vi "Request Data.vi"(6 "Qualifier":string, 8 "error in":errorcluster, 9 "notifier":refnum<notifier>, 10 "Data to Send":string, 11 "MLTFNC in":refnum<class "MLTFNC.lvclass">) -> (0 "error out":errorcluster, 3 "MLTFNC out":refnum<class "MLTFNC.lvclass">)   [LabVIEW 2019, in "MLTFNC.lvlib" / "MLTFNC.lvclass"]
doc: "Data to Send is a required input that describes the measurement or query function to be performed\nQualifier is a secondary variable used in the event that specificity must be provided to the query function\n****Note****\nIf further specificity is required, the qualifier must be used in a comma delimited format to increase the overall variable count. Additional specificity must be provided by the child class and interpreted by the automated call.\n\nnotifier is a single variant notifier in which the instrument will send the data notification to the automated tool."
uses:
  Library/MLTFNC.lvclass
  C:/Users/Public/Documents/Development/builds/Instruments/Instruments.lvlibp/Library/Instruments.lvclass
  builds/Instruments/Instruments.lvlibp/Private/Accessors/Read Poll(ms).vi
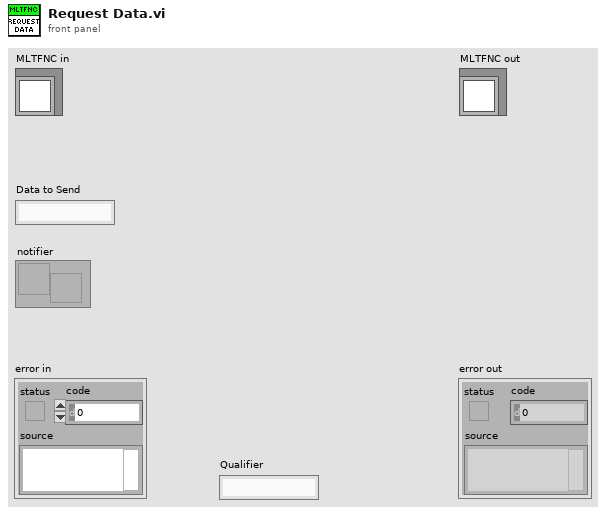
[diagram p1: front panel]
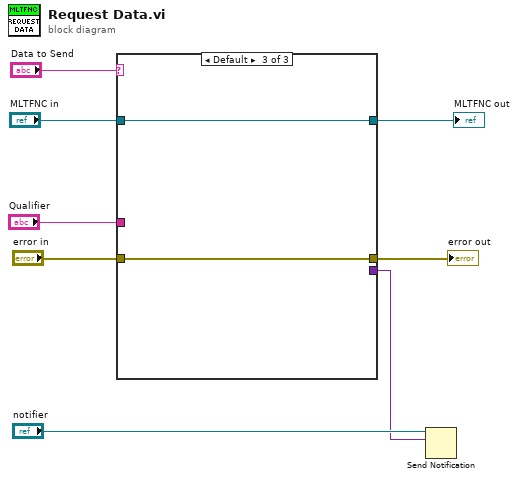
[diagram p0: block diagram]
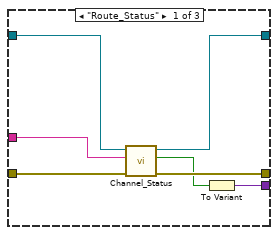
[diagram p2: hidden frame]
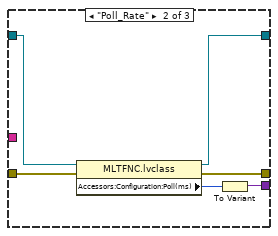
[diagram p3: hidden frame]
diagram:
  n1 = case shown="Default" "Data to Send" {
    tunnel: "MLTFNC in" -> [w15 w19 w23]
    tunnel: [w14 w18 w23] -> w6
    tunnel: "error in" -> [w12 w21 w22]
    tunnel: [w11 w20 w22] -> w3
    tunnel: "Qualifier" -> [w13 _ _]
    tunnel: [w9 w16 _] -> w1
    frame "Route_Status" {
      n2 = call "Channel_Status.vi"("error in"=w12, "Channel"=w13, "MLTFNC in"=w15) -> ("error out"=w11:errorcluster, "Routed"=w10:bool, "MLTFNC out"=w14:refnum<class "MLTFNC.lvclass">)  [unwired: 6 in]
      n3 = To Variant(anything=w10) -> (Variant=w9:variant)
    }
    frame "Poll_Rate" {
      n4 = property class="MLTFNC.lvclass"(reference=w19, error in=w21) -> (reference out=w18:refnum<class "MLTFNC.lvclass">, error out=w20:errorcluster, "Accessors:Configuration:Poll(ms)"=w17:u32)
      n5 = To Variant(anything=w17) -> (Variant=w16:variant)
    }
    frame Default {
    }
  }
  "error out" <- w3
  "MLTFNC out" <- w6
  n6 = Send Notification(notification=w1, notifier="notifier") -> ()  [unwired: 1 in, 2 out]
